vi "Separate_names.vi"   [LabVIEW 2020]
types:
  T1 = cluster{"VIPath":path, "Menu Name":string, "Selector Name":string}[]
  T2 = cluster{"VIPath":path, "Menu Name":string, "Selector Name":string}
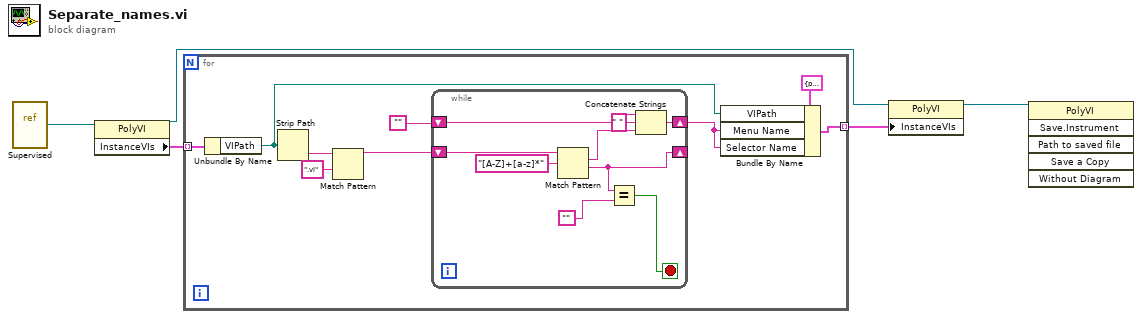
[diagram p0: block diagram]
diagram:
  n1 = vi-ref "Supervised.vi"() -> (w5:refnum<vi>)
  n2 = property class="PolyVI"(reference=w5) -> (reference out=w3:refnum<vi>, "InstanceVIs"=w4:T1)  [unwired: 1 in, 1 out]
  n3 = for {
    tunnel: w4 -> [w14] mode=indexing
    tunnel: [w6] -> w2 mode=indexing
    n4 = Unbundle By Name(w14) -> ("VIPath"=w8:path)
    n5 = Strip Path(path=w8) -> (name=w13:string)  [unwired: 1 out]
    n6 = Match Pattern(string=w13, regular expression=".vi") -> (before substring=w11:string)  [unwired: 1 in, 3 out]
    n7 = while {
      shift-right: [w17] -> _
      shift-left: w11 -> [w23]
      shift-right: [w18] -> w7
      shift-left: "" -> [w19]
      stop <- w15 stop-if-true
      n8 = Match Pattern(string=w23, regular expression="[A-Z]+[a-z]*") -> (match substring=w21:string, after substring=w17:string)  [unwired: 1 in, 2 out]
      n9 = Equal?(x=w17, y="") -> (x = y?=w15:bool)
      n10 = Concatenate Strings(w19, " " ("string"), w21) -> (w18:string)
    }
    n11 = Bundle By Name(cluster=T2 {"VIPath"=path "", "Menu Name"="", "Selector Name"=""} ("input cluster"), "VIPath"=w8, "Menu Name"=w7, "Selector Name"=w7) -> (w6:T2)
  }
  n12 = property class="PolyVI"(reference=w3, "InstanceVIs"=w2) -> (reference out=w1:refnum<vi>)  [unwired: 1 in, 1 out]
  n13 = invoke class="PolyVI" method="Save.Instrument"(reference=w1) -> ()  [unwired: 5 in, 6 out]
